vi "WSVCAP SHL FPGA LL I2C Read Data.vi"(11 "error in (no error)":errorcluster, 13 "Socket Mask":u64 format="%012x") -> (4 "Long Word Out (1-Bit for Each Channel)":u64, 15 "error out":errorcluster)   [LabVIEW 2012]
uses:
  WSVCAP SHL FPGA LL I2C Debug Global.vi
  <vilib>/eio/EIONode/EIONode.xnode
  <vilib>/rvi/eio/common/nirviEmuTemplateMethod_errors.vi
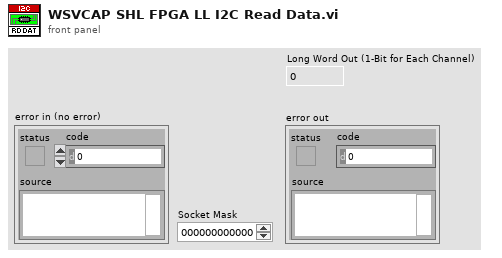
[diagram p1: front panel]
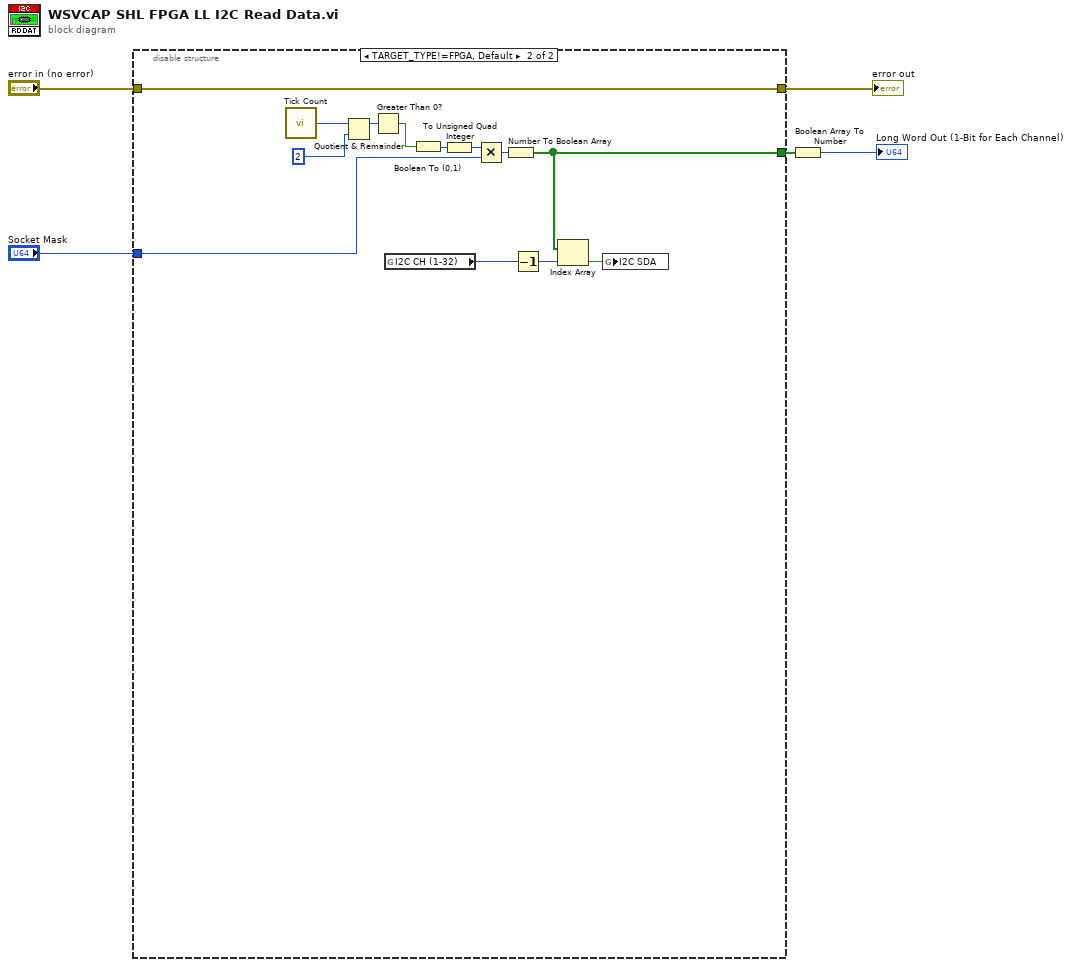
[diagram p0: block diagram]
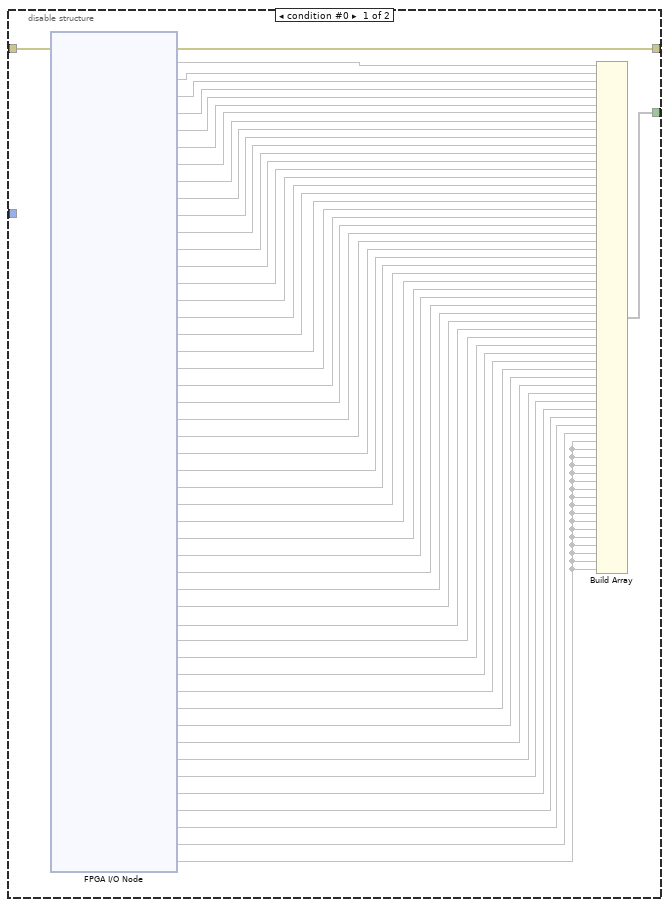
[diagram p2: hidden frame]
diagram:
  n1 = disable-structure shown="TARGET_TYPE!=FPGA, Default" {
    disable-tunnel: [w56 w66] -> w5
    disable-tunnel: "error in (no error)" -> [w55 w66]
    disable-tunnel: "Socket Mask" -> [_ w63]
    disable-tunnel: [w6 w57] -> w1
    frame condition #0 {
      n2 = xnode "FPGA I/O Node"("error in"=w55) -> ("error out"=w56:errorcluster, "I2C_SDA_C1_S1"=w54, "I2C_SDA_C1_S2"=w53, "I2C_SDA_C1_S3"=w52, "I2C_SDA_C1_S4"=w51, "I2C_SDA_C1_S5"=w50, "I2C_SDA_C1_S6"=w49, "I2C_SDA_C1_S7"=w48, "I2C_SDA_C1_S8"=w47, "I2C_SDA_C1_S9"=w46, "I2C_SDA_C1_S10"=w45, "I2C_SDA_C1_S11"=w44, "I2C_SDA_C1_S12"=w43, "I2C_SDA_C1_S13"=w42, "I2C_SDA_C1_S14"=w41, "I2C_SDA_C1_S15"=w40, "I2C_SDA_C1_S16"=w39, "I2C_SDA_C2_S1"=w38, "I2C_SDA_C2_S2"=w37, "I2C_SDA_C2_S3"=w36, "I2C_SDA_C2_S4"=w35, "I2C_SDA_C2_S5"=w34, "I2C_SDA_C2_S6"=w33, "I2C_SDA_C2_S7"=w32, "I2C_SDA_C2_S8"=w31, "I2C_SDA_C2_S9"=w30, "I2C_SDA_C2_S10"=w29, "I2C_SDA_C2_S11"=w28, "I2C_SDA_C2_S12"=w27, "I2C_SDA_C2_S13"=w26, "I2C_SDA_C2_S14"=w25, "I2C_SDA_C2_S15"=w24, "I2C_SDA_C2_S16"=w23, "I2C_SDA_C3_S1"=w22, "I2C_SDA_C3_S2"=w21, "I2C_SDA_C3_S3"=w20, "I2C_SDA_C3_S4"=w19, "I2C_SDA_C3_S5"=w18, "I2C_SDA_C3_S6"=w17, "I2C_SDA_C3_S7"=w16, "I2C_SDA_C3_S8"=w15, "I2C_SDA_C3_S9"=w14, "I2C_SDA_C3_S10"=w13, "I2C_SDA_C3_S11"=w12, "I2C_SDA_C3_S12"=w11, "I2C_SDA_C3_S13"=w10, "I2C_SDA_C3_S14"=w9, "I2C_SDA_C3_S15"=w8, "I2C_SDA_C3_S16"=w7)  [unwired: 48 in, 48 out]
      n3 = Build Array(w54, w53, w52, w51, w50, w49, w48, w47, w46, w45, w44, w43, w42, w41, w40, w39, w38, w37, w36, w35, w34, w33, w32, w31, w30, w29, w28, w27, w26, w25, w24, w23, w22, w21, w20, w19, w18, w17, w16, w15, w14, w13, w12, w11, w10, w9, w8, w7, w7, w7, w7, w7, w7, w7, w7, w7, w7, w7, w7, w7, w7, w7, w7, w7) -> (w6:void[])
    }
    frame condition #1 (active) {
      n4 = call "Tick Count"() -> ("Tick Count(Ticks)"=w69:u32)
      n5 = Quotient & Remainder(x=w69, y=u32 2) -> (x-y*floor(x/y)=w68:u32)  [unwired: 1 out]
      n6 = Greater Than 0?(x=w68) -> (x > 0?=w65:bool)
      n7 = global read "WSVCAP SHL FPGA LL I2C Debug Global.vi" "I2C CH (1-32)"() -> (w62:i32)
      n8 = Boolean To (0,1)(Boolean=w65) -> (0, 1=w64:i16)
      n9 = To Unsigned Quad Integer(1:w64) -> (0:w61:u64)
      n10 = Multiply(x=w61, y=w63) -> (x*y=w60:u64)
      n11 = Number To Boolean Array(number=w60) -> (Boolean array=w57:bool[])
      n12 = Decrement(x=w62) -> (x-1=w58:i32)
      n13 = Index Array(array=w57, index=w58) -> (element=w59:bool)
      n14 = global write "WSVCAP SHL FPGA LL I2C Debug Global.vi" "I2C SDA"(w59) -> ()
    }
  }
  "error out" <- w5
  n15 = Boolean Array To Number(Boolean array=w1) -> (number=→"Long Word Out (1-Bit for Each Channel)":u64)
